vi "Monitor Data Changed.vi"(8 "error in (no error)":errorcluster, 9 "Changed Actor Q":refnum<class "Message Enqueuer.lvclass">, 10 "Monitor Data":refnum<class "Monitor Data.lvclass">, 11 "Classic Actor Monitor in":refnum<class "Classic Monitor.lvclass">) -> (0 "error out":errorcluster, 3 "Classic Actor Monitor out":refnum<class "Classic Monitor.lvclass">)   [LabVIEW 2023, in "Monitored Actor.lvlib" / "Classic Monitor.lvclass"]
doc: "Messages the UI with the new Monitor Data\n\nCopyright: MGI 2016\nAuthor: Derek Trepanier"
uses:
  Classic Monitor.lvclass
  Monitor Data/Monitor Data.lvclass
  builds/Engine/Actor Framework.lvlibp/1abvi3w/vi.lib/ActorFramework/Message Enqueuer/Message Enqueuer.lvclass
  Classic Monitor.lvclass/Classic Monitor.ctl
  Orphan Detector/Orphan Detector Messages/Monitor Stop Msg/Monitor Stop Msg.lvclass
  Logger/Classic Logger Messages/Update Monitor Label Msg/Update Monitor Label Msg.lvclass
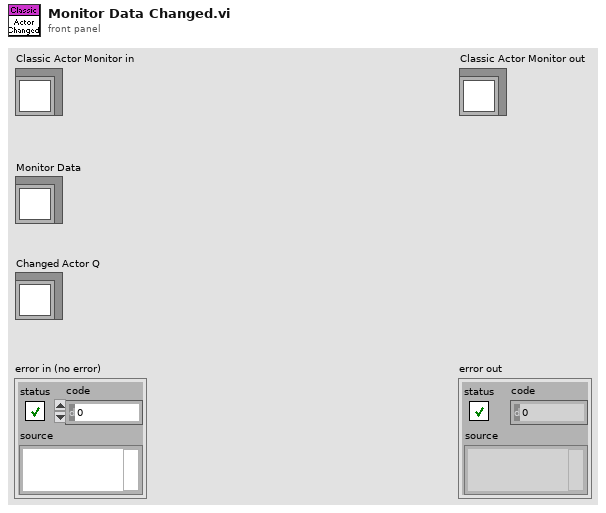
[diagram p1: front panel]
types:
  T1 = typedef "Monitored Actor.lvlib/Monitor Data.lvclass/Actor Data.ctl" = cluster{"Actor Type":string, "Actor Core VI":string, "Self":refnum<class "Message Enqueuer.lvclass">, "Caller":refnum<class "Message Enqueuer.lvclass">, "Actor Label":string, "Last Ping":dbl}
  T2 = cluster{"Monitor Data":refnum<class "Monitor Data.lvclass">, "Changed Actor Q":refnum<class "Message Enqueuer.lvclass">}
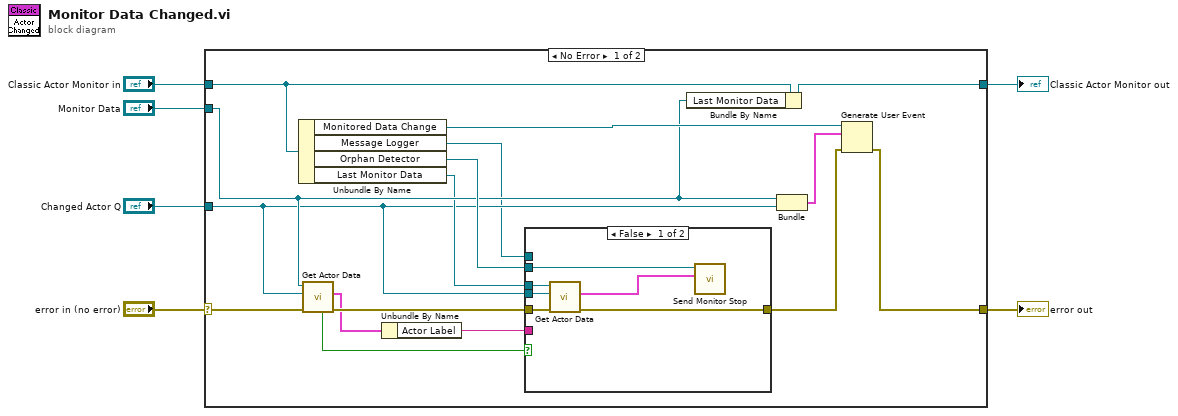
[diagram p0: block diagram]
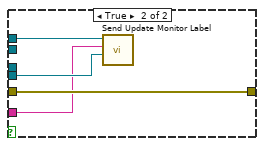
[diagram p2: hidden frame]
diagram:
  n1 = case shown="No Error" "error in (no error)" {
    selector: "error in (no error)" -> [w19 w33]
    tunnel: [w20 w33] -> w6
    tunnel: [w14 w34] -> w5
    tunnel: "Monitor Data" -> [w13 _]
    tunnel: "Classic Actor Monitor in" -> [w22 w34]
    tunnel: "Changed Actor Q" -> [w11 _]
    frame No Error {
      n2 = Unbundle By Name(w22) -> ("Monitored Data Change"=w21:refnum<user-event>, "Message Logger"=w10:refnum<class "Message Enqueuer.lvclass">, "Orphan Detector"=w18:refnum<class "Message Enqueuer.lvclass">, "Last Monitor Data"=w12:refnum<class "Monitor Data.lvclass">)
      n3 = call "Get Actor Data.vi"("error in (no error)"=w19, "Actor's Self Q"=w11, "Monitor Data in"=w13) -> ("error out"=w17:errorcluster, "Actor Data"=w9:T1, "Found?"=w15:bool)  [unwired: 4 in, 2 out]
      n4 = Unbundle By Name(w9) -> ("Actor Label"=w8:string)
      n5 = case shown="False" w15 {
        tunnel: w18 -> [w28 _]
        tunnel: w17 -> [w27 w32]
        tunnel: [w23 w32] -> w16
        tunnel: w12 -> [w25 _]
        tunnel: w11 -> [w24 w30]
        tunnel: w10 -> [_ w31]
        tunnel: w8 -> [_ w29]
        frame False {
          n6 = call "Get Actor Data.vi"("error in (no error)"=w27, "Actor's Self Q"=w24, "Monitor Data in"=w25) -> ("error out"=w23:errorcluster, "Actor Data"=w26:T1)  [unwired: 4 in, 3 out]
          n7 = call "Send Monitor Stop.vi"("Actor Data"=w26, "Message Enqueuer in"=w28) -> ()  [unwired: 8 in, 2 out]
        }
        frame True {
          n8 = call "Send Update Monitor Label.vi"("Actor to Log"=w30, "Label"=w29, "Message Enqueuer in"=w31) -> ()  [unwired: 7 in, 2 out]
        }
      }
      n9 = Bundle By Name(cluster=w22, "Last Monitor Data"=w13) -> (w14:refnum<class "Classic Monitor.lvclass">)
      n10 = Bundle("Monitor Data"=w13, "Changed Actor Q"=w11) -> (w7:T2)  [unwired: 1 in]
      n11 = Generate User Event(user event=w21, event data cluster=w7, error in=w16) -> (error out=w20:errorcluster)  [unwired: 1 in, 1 out]
    }
    frame Error {
    }
  }
  "error out" <- w6
  "Classic Actor Monitor out" <- w5
